vi "Check.vi"(11 "DataIn":T1={"Quem Joga"="", "Tabuleiro"={"(0,0)"="", "(1,0)"="", "(0,1)"="", "(1,1)"="", "(2,0)"="", "(1,2)"="", "(2,2)"="", "(0,2)"="", "(2,1) "=""}, "GameOption"=enum."Multiplayer local", "Turno"=FALSE, "Player"="", "Player 1"="", "Player 2"="", "Dificuldade"=enum."Easy", "Table"=[], "Row"=0, "Aceitar Convite"=FALSE, "Inviter line"=0, "diretório"=path "", "Logout - panel close"=FALSE, "StartGame"=FALSE, "MatchData.lvclass"=refnum, "GameMode"=enum."Single Easy", "Level State"=FALSE}) -> (0 "True = Empatou":bool, 3 "True = Ganhou":bool)   [LabVIEW 2018]
doc: "SubVI criado para checar se houve vitória ou empate através de comparação das posiçõs da matriz do tabuleiro."
uses:
  controls/DataIn.ctl
  MatchDataClasses/MatchData/MatchData.lvclass
  controls/Tabuleiro.ctl
  controls/Table.ctl
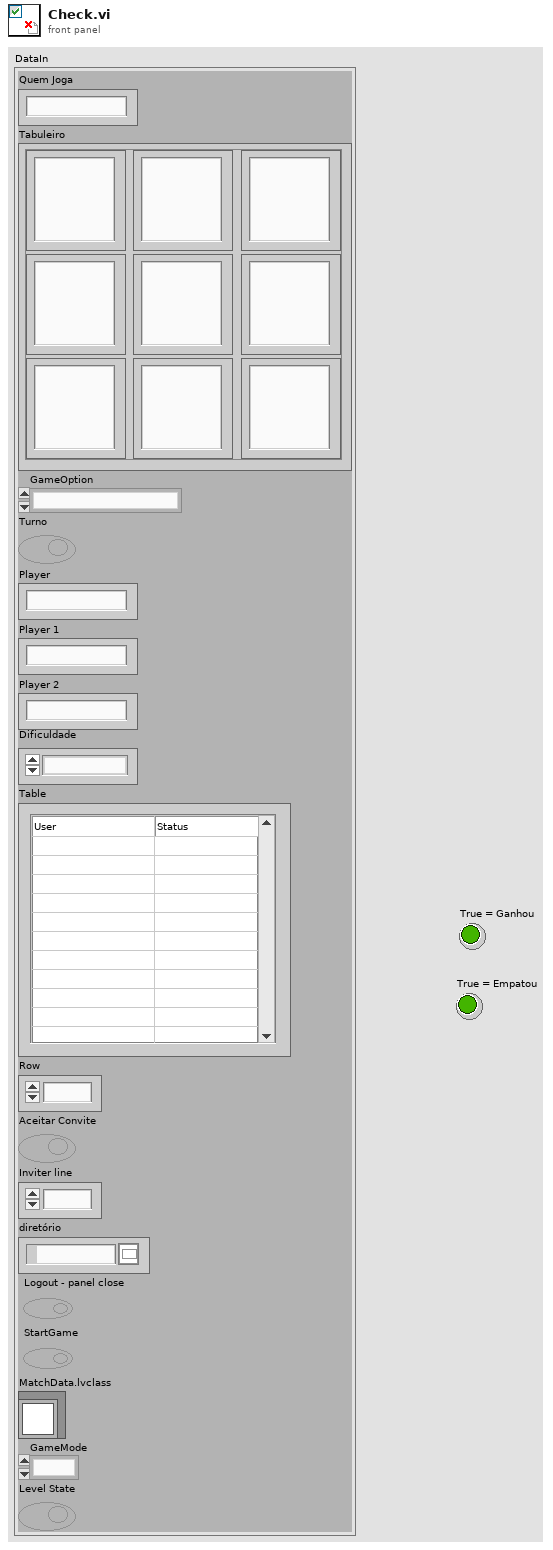
[diagram p1: front panel]
types:
  T1 = typedef "DataIn.ctl" = cluster{"Quem Joga":string, "Tabuleiro":T2, "GameOption":enum16{"Single Player", "Multiplayer local", "Multiplayer remoto", "Wait for Event", "Initialize", "Stop"}, "Turno":bool, "Player":string, "Player 1":string, "Player 2":string, "Dificuldade":enum16{"Easy", "Medium", "Hard"}, "Table":T3, "Row":u32, "Aceitar Convite":bool, "Inviter line":u32, "diretório":path, "Logout - panel close":bool, "StartGame":bool, "MatchData.lvclass":refnum<class "MatchData.lvclass">, "GameMode":enum16{"Single Easy", "Single Medium", "Single Hard", "Local", "Remote"}, "Level State":bool}
  T2 = typedef "Tabuleiro.ctl" = cluster{"(0,0)":string, "(1,0)":string, "(0,1)":string, "(1,1)":string, "(2,0)":string, "(1,2)":string, "(2,2)":string, "(0,2)":string, "(2,1) ":string}
  T3 = typedef "Table.ctl" = string[][]
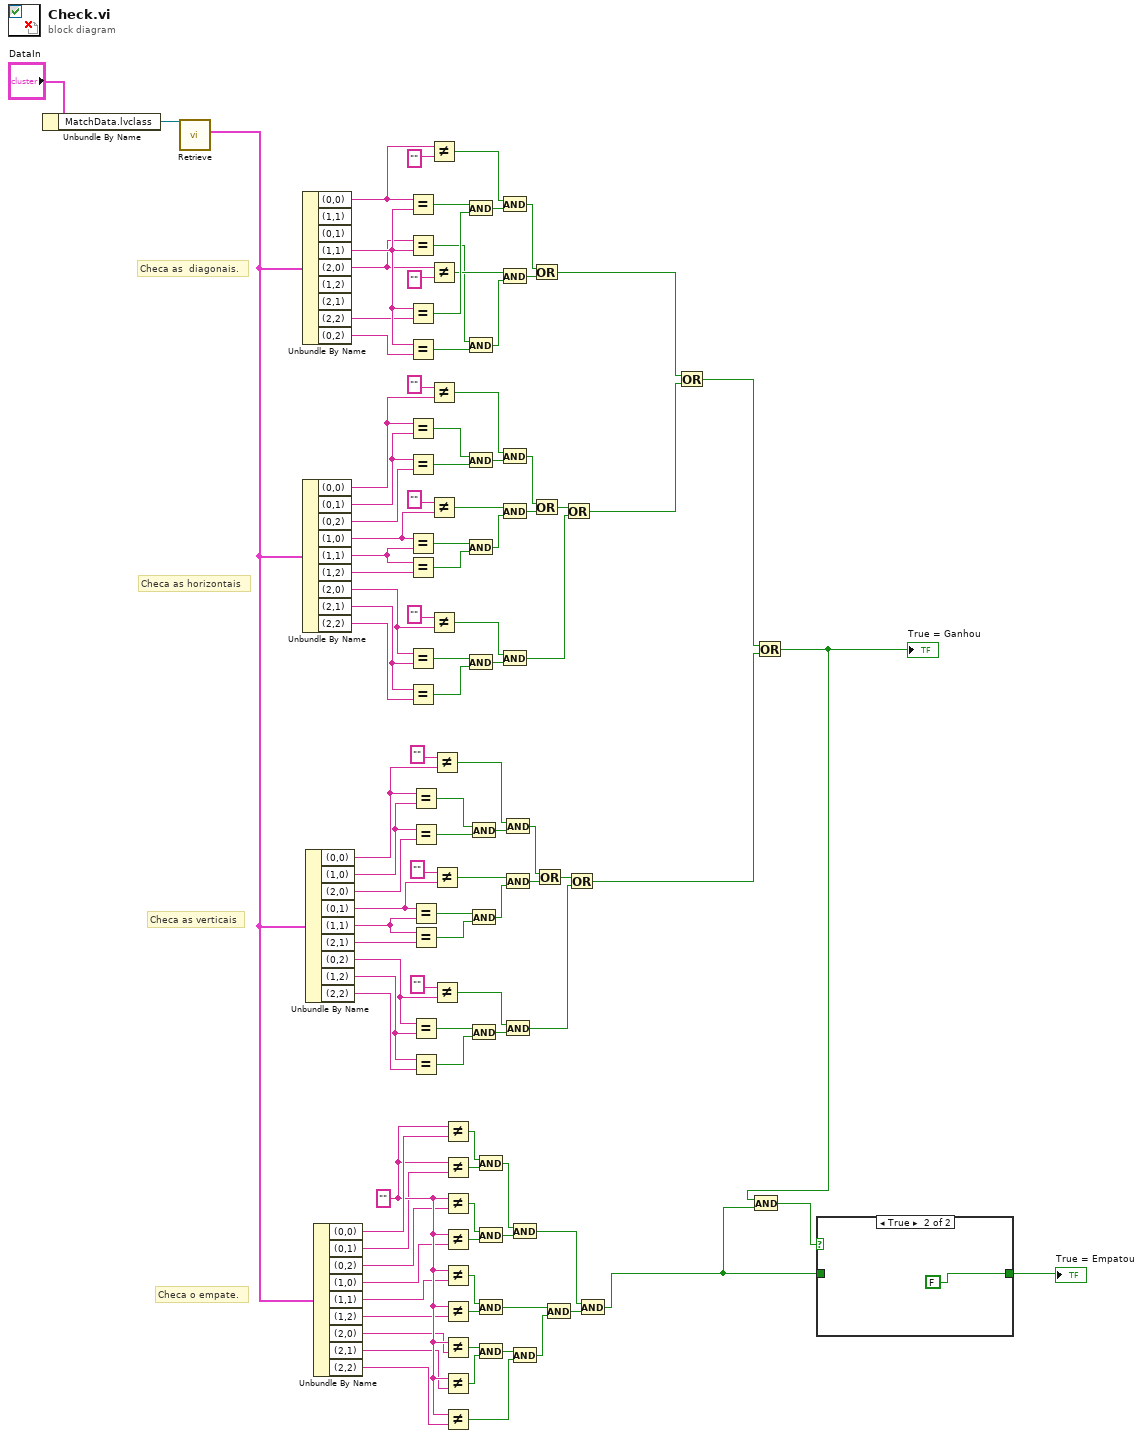
[diagram p0: block diagram]
diagram:
  w33 = "" ("y")
  # "Checa as verticais"
  # "Checa as horizontais"
  # "Checa o empate."
  # "Checa as  diagonais."
  n1 = Unbundle By Name("DataIn") -> ("MatchData.lvclass"=w3:refnum<class "MatchData.lvclass">)
  n2 = call-dynamic "Retrieve.vi"("MatchData in"=w3) -> ("Tabuleiro"=w1:T2)  [unwired: 7 in, 3 out]
  n3 = Unbundle By Name(w1) -> ("(0,0)"=w106:string, "(1,1)"=w109:string, "(2,0)"=w108:string, "(2,2)"=w107:string, "(0,2)"=w110:string)  [unwired: 4 out]
  n4 = Unbundle By Name(w1) -> ("(0,0)"=w92:string, "(0,1)"=w91:string, "(0,2)"=w90:string, "(1,0)"=w84:string, "(1,1)"=w83:string, "(1,2)"=w82:string, "(2,0)"=w76:string, "(2,1)"=w74:string, "(2,2)"=w75:string)
  n5 = Unbundle By Name(w1) -> ("(0,0)"=w64:string, "(1,0)"=w63:string, "(2,0)"=w62:string, "(0,1)"=w56:string, "(1,1)"=w55:string, "(2,1)"=w54:string, "(0,2)"=w48:string, "(1,2)"=w46:string, "(2,2)"=w47:string)
  n6 = Unbundle By Name(w1) -> ("(0,0)"=w34:string, "(0,1)"=w32:string, "(0,2)"=w31:string, "(1,0)"=w30:string, "(1,1)"=w29:string, "(1,2)"=w28:string, "(2,0)"=w27:string, "(2,1)"=w26:string, "(2,2)"=w4:string)
  n7 = Equal?(x=w106, y=w109) -> (x = y?=w101:bool)
  n8 = Equal?(x=w108, y=w109) -> (x = y?=w97:bool)
  n9 = Equal?(x=w109, y=w107) -> (x = y?=w100:bool)
  n10 = Equal?(x=w109, y=w110) -> (x = y?=w96:bool)
  n11 = Equal?(x=w92, y=w91) -> (x = y?=w89:bool)
  n12 = Equal?(x=w91, y=w90) -> (x = y?=w88:bool)
  n13 = Equal?(x=w84, y=w83) -> (x = y?=w81:bool)
  n14 = Equal?(x=w83, y=w82) -> (x = y?=w80:bool)
  n15 = Equal?(x=w76, y=w74) -> (x = y?=w73:bool)
  n16 = Equal?(x=w74, y=w75) -> (x = y?=w72:bool)
  n17 = Equal?(x=w64, y=w63) -> (x = y?=w61:bool)
  n18 = Equal?(x=w63, y=w62) -> (x = y?=w60:bool)
  n19 = Equal?(x=w56, y=w55) -> (x = y?=w53:bool)
  n20 = Equal?(x=w55, y=w54) -> (x = y?=w52:bool)
  n21 = Equal?(x=w48, y=w46) -> (x = y?=w45:bool)
  n22 = Equal?(x=w46, y=w47) -> (x = y?=w44:bool)
  n23 = Not Equal?(x=w106, y="") -> (x != y?=w103:bool)
  n24 = Not Equal?(x=w108, y="") -> (x != y?=w98:bool)
  n25 = Not Equal?(x="" ("y"), y=w92) -> (x != y?=w87:bool)
  n26 = Not Equal?(x="" ("y"), y=w84) -> (x != y?=w78:bool)
  n27 = Not Equal?(x="" ("y"), y=w76) -> (x != y?=w70:bool)
  n28 = Not Equal?(x="" ("y"), y=w64) -> (x != y?=w59:bool)
  n29 = Not Equal?(x="" ("y"), y=w56) -> (x != y?=w50:bool)
  n30 = Not Equal?(x="" ("y"), y=w48) -> (x != y?=w42:bool)
  n31 = Not Equal?(x=w33, y=w34) -> (x != y?=w25:bool)
  n32 = Not Equal?(x=w33, y=w32) -> (x != y?=w24:bool)
  n33 = Not Equal?(x=w33, y=w31) -> (x != y?=w23:bool)
  n34 = Not Equal?(x=w33, y=w30) -> (x != y?=w22:bool)
  n35 = Not Equal?(x=w33, y=w29) -> (x != y?=w21:bool)
  n36 = Not Equal?(x=w33, y=w28) -> (x != y?=w20:bool)
  n37 = Not Equal?(x=w33, y=w27) -> (x != y?=w19:bool)
  n38 = Not Equal?(x=w33, y=w26) -> (x != y?=w18:bool)
  n39 = Not Equal?(x=w33, y=w4) -> (x != y?=w17:bool)
  n40 = And(x=w101, y=w100) -> (x .and. y?=w102:bool)
  n41 = And(x=w97, y=w96) -> (x .and. y?=w99:bool)
  n42 = And(x=w89, y=w88) -> (x .and. y?=w86:bool)
  n43 = And(x=w81, y=w80) -> (x .and. y?=w79:bool)
  n44 = And(x=w73, y=w72) -> (x .and. y?=w71:bool)
  n45 = And(x=w61, y=w60) -> (x .and. y?=w58:bool)
  n46 = And(x=w53, y=w52) -> (x .and. y?=w51:bool)
  n47 = And(x=w45, y=w44) -> (x .and. y?=w43:bool)
  n48 = And(x=w25, y=w24) -> (x .and. y?=w13:bool)
  n49 = And(x=w23, y=w22) -> (x .and. y?=w12:bool)
  n50 = And(x=w21, y=w20) -> (x .and. y?=w14:bool)
  n51 = And(x=w19, y=w18) -> (x .and. y?=w16:bool)
  n52 = And(x=w103, y=w102) -> (x .and. y?=w104:bool)
  n53 = And(x=w98, y=w99) -> (x .and. y?=w105:bool)
  n54 = And(x=w87, y=w86) -> (x .and. y?=w69:bool)
  n55 = And(x=w78, y=w79) -> (x .and. y?=w68:bool)
  n56 = And(x=w70, y=w71) -> (x .and. y?=w67:bool)
  n57 = And(x=w59, y=w58) -> (x .and. y?=w41:bool)
  n58 = And(x=w50, y=w51) -> (x .and. y?=w40:bool)
  n59 = And(x=w42, y=w43) -> (x .and. y?=w39:bool)
  n60 = And(x=w13, y=w12) -> (x .and. y?=w11:bool)
  n61 = And(x=w16, y=w17) -> (x .and. y?=w15:bool)
  n62 = Or(x=w104, y=w105) -> (x .or. y?=w37:bool)
  n63 = Or(x=w69, y=w68) -> (x .or. y?=w66:bool)
  n64 = Or(x=w41, y=w40) -> (x .or. y?=w38:bool)
  n65 = And(x=w14, y=w15) -> (x .and. y?=w10:bool)
  n66 = Or(x=w66, y=w67) -> (x .or. y?=w36:bool)
  n67 = Or(x=w38, y=w39) -> (x .or. y?=w9:bool)
  n68 = And(x=w11, y=w10) -> (x .and. y?=w8:bool)
  n69 = Or(x=w37, y=w36) -> (x .or. y?=w35:bool)
  n70 = Or(x=w35, y=w9) -> (x .or. y?=w5:bool)
  "True = Ganhou" <- w5
  n71 = And(x=w5, y=w8) -> (x .and. y?=w7:bool)
  n72 = case shown="True" w7 {
    tunnel: w8 -> [w111 _]
    tunnel: [w111 FALSE] -> w6
    frame False {
    }
    frame True {
    }
  }
  "True = Empatou" <- w6
